vi "Check Boundary Collisions.vi"(6 "Lower Boundary":dbl, 9 "Upper Boundary":i16, 10 "Velocity":dbl, 11 "Position":dbl) -> (2 "Hit Lower Boundary?":bool, 3 "Hit Upper Boundary?":bool)   [LabVIEW 2015]
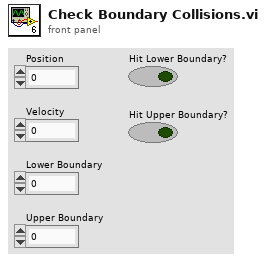
[diagram p1: front panel]
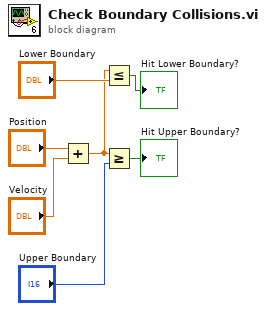
[diagram p0: block diagram]
diagram:
  n1 = Add(x="Position", y="Velocity") -> (x+y=w3:dbl)
  n2 = Less Or Equal?(x=w3, y="Lower Boundary") -> (x <= y?=→"Hit Lower Boundary?":bool)
  n3 = Greater Or Equal?(x=w3, y="Upper Boundary") -> (x >= y?=→"Hit Upper Boundary?":bool)
